vi "Configure TV Trigger Source [TV].vi"(0 "CS++Scope":refnum<class "CS++Scope.lvclass">, 1 "trigger source (\"CHANNEL1\")":string(combo)="CHANNEL1", 2 "tv event (Field 1)":i32(ring)=1 items=["Field 1"=1, "Field 2"=2, "Any Field"=3, "Any Line"=4, "Line Number"=5], 3 "tv trigger polarity (Positive)":i32(ring)=1 items=["Positive"=1, "Negative"=2], 4 "tv signal format (NTSC)":i32(ring)=1 items=["NTSC"=1, "PAL"=2, "SECAM"=3], 5 "error in (no error)":errorcluster) -> (14 "CS++Scope out":refnum<class "CS++Scope.lvclass">, 19 "error out":errorcluster)   [LabVIEW 2013, in "CS++Scope.lvlib" / "CS++Scope.lvclass"]
doc: "This VI configures the oscilloscope for TV triggering. It configures the TV signal format, the event and the signal polarity."
uses:
  CS++Scope.lvclass
  CSPP_Core/Classes/CS++ProcessVariables/ProcessVariable/PV.lvclass
  PV-Enum.ctl
  CS++Scope.lvclass/CS++Scope.ctl
  CSPP_Core/Classes/CS++ProcessVariables/PVConnection/PVConnection.lvclass
  CSPP_Core/Classes/CS++ProcessVariables/ProcessVariable/PV.lvclass/PV.ctl
  CSPP_Core/Classes/CS++ProcessVariables/ProcessVariable/Write Data.vi
  CSPP_Core/Classes/CS++ProcessVariables/ProcessVariable/Write Timestamp.vi
  CSPP_Core/Classes/CS++ProcessVariables/ProcessVariable/Write Quality.vi
  CSPP_Core/Classes/CS++ProcessVariables/ProcessVariable/Write status.vi
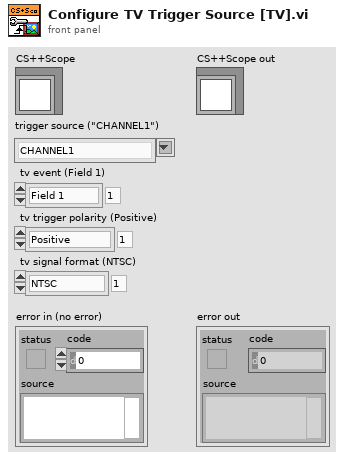
[diagram p1: front panel]
types:
  T1 = typedef "CS++Scope.lvlib/CS++Scope.lvclass/PV-Enum.ctl" = enum16{"ActualSampleRate", "TimePerRecord", "AcquisitionStartTime", "TriggerLevel", "GlitchWidth", "LowReference", "MidReference", "HighReference", "RuntLowThreshold", "RuntHighThreshold", "TriggerHoldoff", "WidthLowThreshold", "WidthHighThreshold", "AcquisitionStatus", "ActualRecordLength", "ActualSampleMode", "ACLineTriggerSlope", "MinRecordLength", "AcquisitionType", "TriggerSlope", "GlitchCondition", "GlitchPolarity", "InterpolationMethod", "NumberOfAverages", "NumberOfEnvelopes", "TriggerType", "TriggerCoupling", "TriggerModifier", "TVLineNumber", "TVEvent", "TVTriggerPolarity", "TVSignalFormat", "WidthCondition", "WidthPolarity", "MeasurementDone", "ContinousAcquisition", "TriggerSource", "Waveform"}
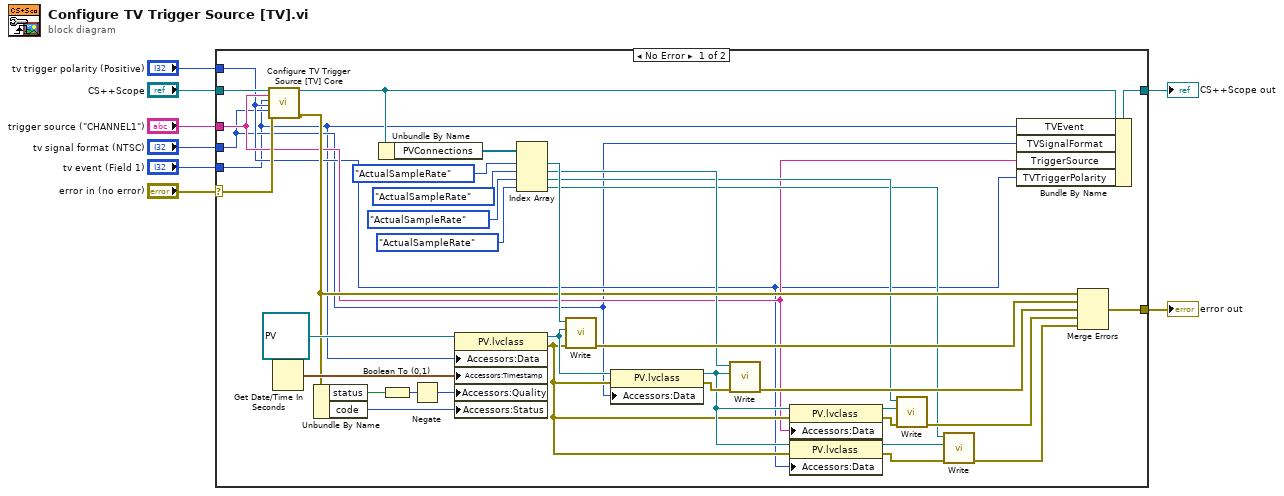
[diagram p0: block diagram]
diagram:
  n1 = case shown="No Error" "error in (no error)" {
    selector: "error in (no error)" -> [w13 w47]
    tunnel: [w14 w47] -> w7
    tunnel: [w15 w46] -> w2
    tunnel: "CS++Scope" -> [w16 w46]
    tunnel: "trigger source (\"CHANNEL1\")" -> [w12 _]
    tunnel: "tv signal format (NTSC)" -> [w10 _]
    tunnel: "tv event (Field 1)" -> [w9 _]
    tunnel: "tv trigger polarity (Positive)" -> [w11 _]
    frame No Error {
      n2 = call-dynamic "Configure TV Trigger Source [TV] Core.vi"("CS++Scope"=w16, "trigger source (\"CHANNEL1\")"=w12, "tv event (Field 1)"=w9, "tv trigger polarity (Positive)"=w11, "tv signal format (NTSC)"=w10, "error in (no error)"=w13) -> ("CS++Scope out"=w35:refnum<class "CS++Scope.lvclass">, "error out"=w34:errorcluster)  [unwired: 12 in]
      n3 = Get Date/Time In Seconds() -> (seconds since 1Jan1904=w40:timestamp)
      n4 = Unbundle By Name(w34) -> ("status"=w43:bool, "code"=w44:i32)
      n5 = Unbundle By Name(w35) -> ("PVConnections"=w39:refnum<class "PVConnection.lvclass">[])
      n6 = Boolean To (0,1)(Boolean=w43) -> (0, 1=w42:i16)
      n7 = Negate(x=w42) -> (-x=w41:i16)
      n8 = property class="PV.lvclass"(reference=refnum<class "PV.lvclass"> refnum ("CS++ProcessVariables.lvlib:PV.lvclass"), "Accessors:Data"=w9, "Accessors:Timestamp"=w40, "Accessors:Quality"=w41, "Accessors:Status"=w44) -> (reference out=w29:refnum<class "PV.lvclass">, error out=w18:errorcluster)  [unwired: 1 in]
      n9 = Index Array(array=w39, index #1=PV-Enum."ActualSampleRate" ("PV-Enum"), index #2=PV-Enum."ActualSampleRate" ("PV-Enum"), index #3=PV-Enum."ActualSampleRate" ("PV-Enum"), index #4=PV-Enum."ActualSampleRate" ("PV-Enum")) -> (element #1=w37:refnum<class "PVConnection.lvclass">, element #2=w27:refnum<class "PVConnection.lvclass">, element #3=w25:refnum<class "PVConnection.lvclass">, element #4=w20:refnum<class "PVConnection.lvclass">)
      n10 = call-dynamic "Write.vi"("error in (no error)"=w18, "PV"=w29, "PVConnection in"=w37) -> ("error out"=w36:errorcluster)  [unwired: 7 in, 1 out]
      n11 = property class="PV.lvclass"(reference=w29, error in=w18, "Accessors:Data"=w10) -> (reference out=w19:refnum<class "PV.lvclass">, error out=w28:errorcluster)
      n12 = call-dynamic "Write.vi"("error in (no error)"=w28, "PV"=w19, "PVConnection in"=w27) -> ("error out"=w31:errorcluster)  [unwired: 7 in, 1 out]
      n13 = property class="PV.lvclass"(reference=w19, error in=w18, "Accessors:Data"=w12) -> (reference out=w26:refnum<class "PV.lvclass">, error out=w24:errorcluster)
      n14 = property class="PV.lvclass"(reference=w19, error in=w18, "Accessors:Data"=w11) -> (reference out=w22:refnum<class "PV.lvclass">, error out=w21:errorcluster)
      n15 = call-dynamic "Write.vi"("error in (no error)"=w24, "PV"=w26, "PVConnection in"=w25) -> ("error out"=w30:errorcluster)  [unwired: 7 in, 1 out]
      n16 = call-dynamic "Write.vi"("error in (no error)"=w21, "PV"=w22, "PVConnection in"=w20) -> ("error out"=w17:errorcluster)  [unwired: 7 in, 1 out]
      n17 = Bundle By Name(cluster=w35, "TVEvent"=w9, "TVSignalFormat"=w10, "TriggerSource"=w12, "TVTriggerPolarity"=w11) -> (w15:refnum<class "CS++Scope.lvclass">)
      n18 = Merge Errors(w34, w36, w31, w30, w17) -> (w14:errorcluster)
    }
    frame Error {
    }
  }
  "error out" <- w7
  "CS++Scope out" <- w2
